vi "Local_Read_INI_Sub_VI_SM.vi"(11 "Config File Path":path) -> (3 "output cluster":T1)   [LabVIEW 2017]
uses:
  <vilib>/Utility/config.llb/Read Key (Path).vi
  <vilib>/Utility/config.llb/Read Key (I32).vi
  <vilib>/Utility/config.llb/Read Key (String).vi
  <vilib>/Utility/config.llb/NI_LVConfig.lvlib
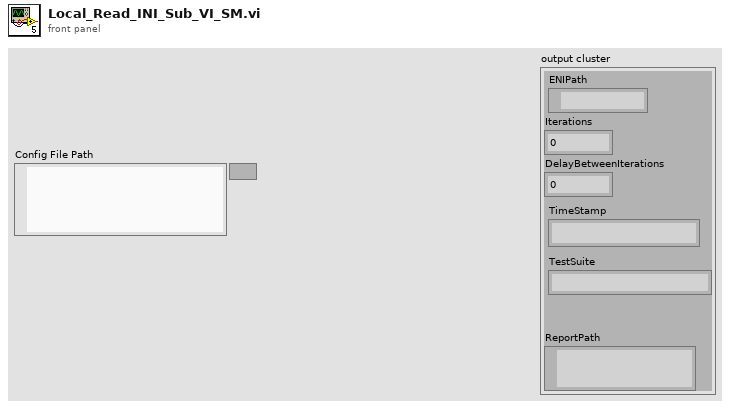
[diagram p1: front panel]
types:
  T1 = cluster{"ENIPath":path, "Iterations":i32, "DelayBetweenIterations":i32, "TimeStamp":string, "TestSuite":string, "ReportPath":path}
  T2 = typedef "NI_LVConfig.lvlib/Config Data RefNum.ctl" = refnum<k1>
  T3 = cluster{"value":path, "value":i32, "value":i32, "value":string, "default value":string, "value":path}
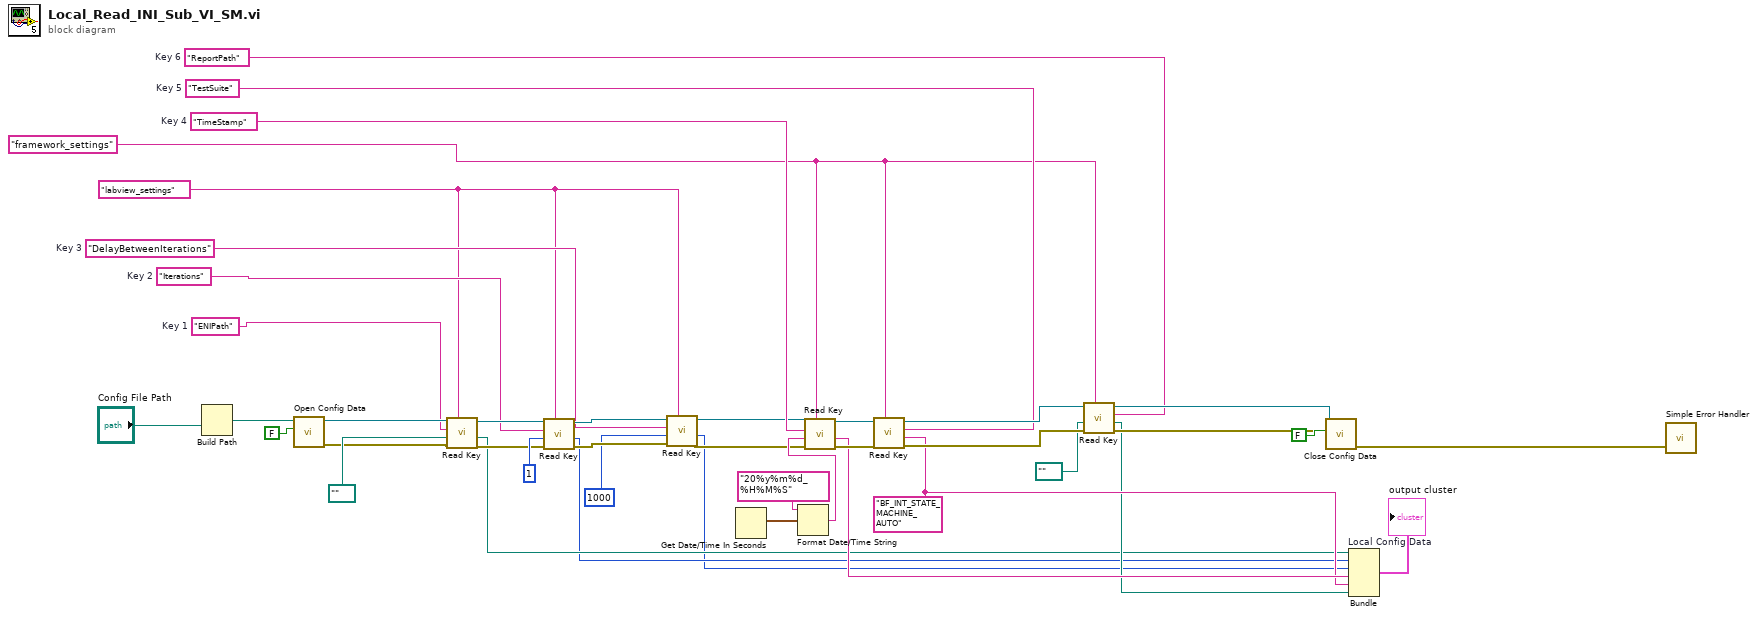
[diagram p0: block diagram]
diagram:
  w1 = "labview_settings" ("section")
  w7 = "ENIPath"  # Key 1
  w9 = "DelayBetweenIterations"  # Key 3
  w8 = "Iterations"  # Key 2
  w23 = "TimeStamp"  # Key 4
  w20 = "BF_INT_STATE_MACHINE_AUTO" ("default value")
  w31 = "TestSuite"  # Key 5
  w34 = "ReportPath"  # Key 6
  w2 = "framework_settings" ("section")
  n1 = Build Path(name or relative path="Config File Path") -> (appended path=w38:path)  [unwired: 1 in]
  n2 = call <vilib>:"Open Config Data.vi"("create file if necessary (T)"=FALSE ("create file if necessary? (T)"), "configuration file path"=w38) -> ("error out"=w29:errorcluster, "refnum"=w28:T2)  [unwired: 7 in, 1 out]
  n3 = call-poly <vilib>:"Read Key.vi"("section"=w1, "error in (no error)"=w29, "default value"=path "", "key"=w7, "refnum"=w28) -> ("error out"=w12:errorcluster, "value"=w6:path, "refnum out"=w13:T2)  [unwired: 1 in, 3 out]
  n4 = call-poly <vilib>:"Read Key.vi"("section"=w1, "error in (no error)"=w12, "default value"=1, "key"=w8, "refnum"=w13) -> ("error out"=w16:errorcluster, "value"=w5:i32, "refnum out"=w17:T2)  [unwired: 4 out]
  n5 = call-poly <vilib>:"Read Key.vi"("section"=w1, "error in (no error)"=w16, "default value"=1000, "key"=w9, "refnum"=w17) -> ("error out"=w10:errorcluster, "value"=w4:i32, "refnum out"=w11:T2)  [unwired: 4 out]
  n6 = Get Date/Time In Seconds() -> (seconds since 1Jan1904=w26:timestamp)
  n7 = Format Date/Time String(time format string (%c)="20%y%m%d_%H%M%S", seconds (now)=w26) -> (date/time string=w22:string)  [unwired: 1 out]
  n8 = call-poly <vilib>:"Read Key.vi"("section"=w2, "error in (no error)"=w10, "default value"=w22, "key"=w23, "refnum"=w11) -> ("error out"=w25:errorcluster, "value"=w21:string, "refnum out"=w24:T2)  [unwired: 1 in, 3 out]
  n9 = call-poly <vilib>:"Read Key.vi"("section"=w2, "error in (no error)"=w25, "default value"=w20, "key"=w31, "refnum"=w24) -> ("error out"=w32:errorcluster, "refnum out"=w33:T2)  [unwired: 1 in, 4 out]
  n10 = call-poly <vilib>:"Read Key.vi"("section"=w2, "error in (no error)"=w32, "default value"=path "", "key"=w34, "refnum"=w33) -> ("error out"=w35:errorcluster, "value"=w19:path, "refnum out"=w36:T2)  [unwired: 1 in, 3 out]
  n11 = call <vilib>:"Close Config Data.vi"("error in (no error)"=w35, "write file if changed (T)"=FALSE ("write configuration file? (T)"), "refnum"=w36) -> ("error out"=w39:errorcluster)  [unwired: 8 out]
  n12 = Bundle "Local Config Data"("value"=w6, "value"=w5, "value"=w4, "value"=w21, "default value"=w20, "value"=w19) -> (→"output cluster":T3)  [unwired: 1 in]
  n13 = call <vilib>:"Simple Error Handler.vi"("error in (no error)"=w39) -> ()  [unwired: 1 in, 8 out]
